vi "serial 클러스터.vi"() -> ()   [LabVIEW 2014]
uses:
  <vilib>/Instr/_visa.llb/VISA Configure Serial Port (Instr).vi
panel:
  in  "serial":T1={"VISA resource name"="", "baud rate (9600)"=9600, "data bits (8)"=8, "parity (0:none)"=enum."None", "error in (no error)"={"status"=FALSE, "code"=0, "source"=""}} {"data bits (8)" min=5 max=8 step=1}
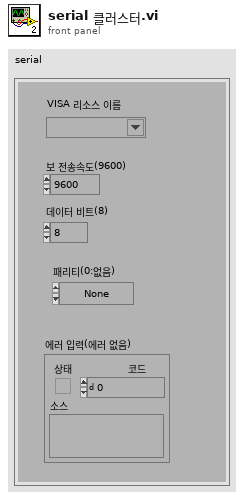
[diagram p1: front panel]
types:
  T1 = cluster{"VISA resource name":refnum<visa-resource-name>, "baud rate (9600)":u32, "data bits (8)":u16, "parity (0:none)":enum16{"None", "Odd", "Even", "Mark", "Space"}, "error in (no error)":errorcluster}
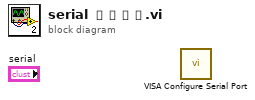
[diagram p0: block diagram]
diagram:
  n1 = call-poly "VISA Configure Serial Port"() -> ()  [unwired: 14 in, 2 out]
